vi "Transaction ID.vi"() -> (2 "Transaction ID":u16)   [LabVIEW 2021, in "IP Data Unit.lvclass"]
uses:
  IP Data Unit.lvclass
  IP Data Unit.lvclass/IP Data Unit.ctl
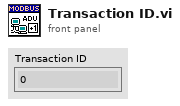
[diagram p1: front panel]
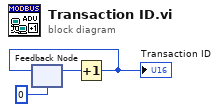
[diagram p0: block diagram]
diagram:
  n1 = feedback #1(u16 0) -> (w2:u16)
  n2 = Increment(x=w2) -> (x+1=w1:u16)
  "Transaction ID" <- w1
  n3 = feedback-in #1(w1) -> ()
